vi "ws_configure restart dynamic.vi"() -> ()   [LabVIEW 2011]
panel:
  in  "rendezvous":T1
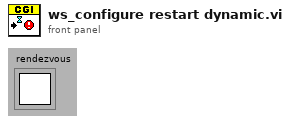
[diagram p1: front panel]
types:
  T1 = typedef "Rendezvous RefNum" = refnum<k1>
  T2 = typedef "Keyed Array.ctl" = cluster{"keys":string[], "values":string[]}
  T3 = enum32{"invalid app kind", "Development System", "Run Time System", "Student Edition", "Embedded LabVIEW", "Evaluation", "Custom"}
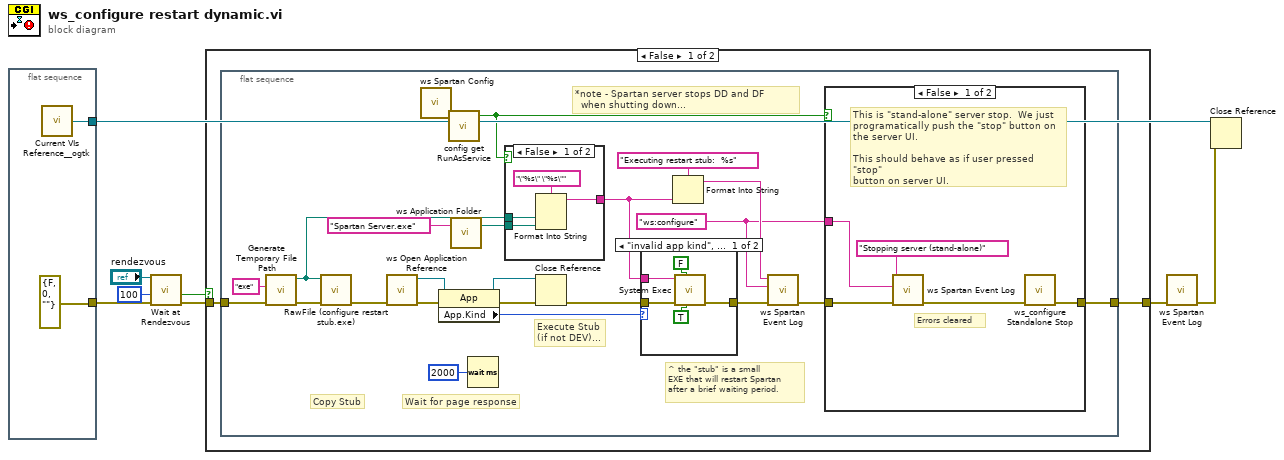
[diagram p0: block diagram]
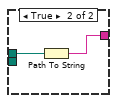
[diagram p2: hidden frame]
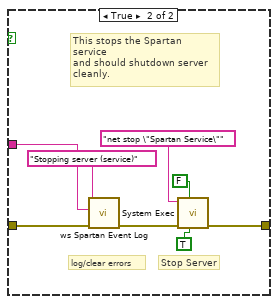
[diagram p4: hidden frame]
diagram:
  n1 = flat-sequence {
    tunnel: [w9] -> w3
    tunnel: [errorcluster {"status"=FALSE, "code"=0, "source"=""} ("error in (no error)")] -> w4
    frame #0 {
      n2 = call <userlib>:"Current VIs Reference__ogtk.vi"() -> ("Current VI's reference"=w9:refnum<vi>)  [unwired: 5 out]
    }
  }
  n3 = call <vilib>:"Wait at Rendezvous.vi"("error in (no error)"=w4, "ms timeout (-1)"=100, "rendezvous"="rendezvous") -> ("error out"=w6:errorcluster, "timed out"=w5:bool)  [unwired: 3 out]
  n4 = case shown="False" w5 {
    tunnel: [w12 w61] -> w2
    tunnel: w6 -> [w11 w61]
    frame False {
      n5 = flat-sequence {
        tunnel: [w35] -> w12
        tunnel: w11 -> [w19]
        frame #0 {
          w30 = "ws:configure" ("command line")
          # "Wait for page response"
          # "Copy Stub"
          # "*note - Spartan server stops DD and DF\n  when shutting down..."
          # "^ the \"stub\" is a small\nEXE that will restart Spartan\nafter a brief waiting period."
          # "Execute Stub\n(if not DEV)..."
          n6 = call <vilib>:"Generate Temporary File Path.vi"("error in (no error)"=w19, "Temporary File Extension (tmp)"="exe") -> ("error out"=w23:errorcluster, "Unique Temporary File Path"=w20:path)  [unwired: 8 out]
          n7 = call "RawFile (configure restart stub.exe).vi"("error in (no error)"=w23, "Path to File (empty)"=w20) -> ("error out"=w15:errorcluster)  [unwired: 9 out]
          n8 = call "ws Open Application Reference.vi"("error in (no error)"=w15) -> ("error out"=w14:errorcluster, "application reference"=w13:refnum<vi>)  [unwired: 9 in]
          n9 = call "ws Spartan Config.vi"() -> ("CONFIG"=w16:T2)  [unwired: 9 in, 2 out]
          n10 = property class="App"(reference=w13, error in=w14) -> (reference out=w25:refnum<vi>, error out=w26:errorcluster, "App.Kind"=w27:T3)
          n11 = call "config get RunAsService.vi"("Config Keys"=w16) -> ("RunAsService?"=w34:bool)  [unwired: 4 out]
          n12 = call "ws Application Folder.vi"("Relative Path (\"\" - Folder)"="Spartan Server.exe" ("command line")) -> ("Application Folder"=w17:path)  [unwired: 2 in]
          n13 = Wait (ms)(milliseconds to wait=u32 2000) -> ()  [unwired: 1 out]
          n14 = case shown="False" w34 {
            tunnel: [w38 w40] -> w31
            tunnel: w20 -> [w37 w41]
            tunnel: w17 -> [w36 _]
            frame False {
              n15 = Format Into String(format string="\"%s\" \"%s\"", w37, w36) -> (resulting string=w38:string)  [unwired: 2 in, 1 out]
            }
            frame True {
              n16 = Path To String(path=w41) -> (string=w40:string)
            }
          }
          n17 = Close Reference(reference=w25, error in (no error)=w26) -> (error out=w24:errorcluster)
          n18 = case shown="\"invalid app kind\", Default" w27 {
            tunnel: w24 -> [w44 w47]
            tunnel: [w43 w47] -> w29
            tunnel: w31 -> [w42 _]
            frame "invalid app kind", Default {
              n19 = call <vilib>:"System Exec.vi"("run minimized? (F)"=TRUE, "wait until completion? (T)"=FALSE, "error in (no error)"=w44, "command line"=w42) -> ("error out"=w43:errorcluster)  [unwired: 2 in, 5 out]
            }
            frame "Development System" {
            }
          }
          n20 = Format Into String(format string="Executing restart stub:  %s", w31) -> (resulting string=w32:string)  [unwired: 2 in, 1 out]
          n21 = call "ws Spartan Event Log.vi"("error in (no error)"=w29, "module (\"\")"=w30, "message (\"\")"=w32) -> ("error out"=w28:errorcluster)  [unwired: 5 in]
          n22 = case shown="False" w34 {
            tunnel: w28 -> [w52 w53]
            tunnel: [w48 w58] -> w35
            tunnel: w30 -> [w51 w54]
            frame False {
              # "Errors cleared"
              # "This is \"stand-alone\" server stop.  We just\nprogramatically push the \"stop\" button on\nthe server UI.\n\nThis should behave as if user pressed \"stop\"\nbutton on server UI."
              n23 = call "ws Spartan Event Log.vi"("error in (no error)"=w52, "module (\"\")"=w51, "message (\"\")"="Stopping server (stand-alone)") -> ("error out"=w49:errorcluster)  [unwired: 5 in]
              n24 = call "ws_configure Standalone Stop.vi"("error in (no error)"=w49) -> ("error out"=w48:errorcluster)  [unwired: 6 in]
            }
            frame True {
              # "This stops the Spartan service\nand should shutdown server\ncleanly."
              # "Stop Server"
              # "log/clear errors"
              n25 = call "ws Spartan Event Log.vi"("error in (no error)"=w53, "module (\"\")"=w54, "message (\"\")"="Stopping server (service)") -> ("error out"=w56:errorcluster)  [unwired: 5 in]
              n26 = call <vilib>:"System Exec.vi"("run minimized? (F)"=TRUE, "wait until completion? (T)"=FALSE, "error in (no error)"=w56, "command line"="net stop \"Spartan Service\"") -> ("error out"=w58:errorcluster)  [unwired: 2 in, 5 out]
            }
          }
        }
      }
    }
    frame True {
    }
  }
  n27 = call "ws Spartan Event Log.vi"("error in (no error)"=w2) -> ("error out"=w1:errorcluster)  [unwired: 7 in]
  n28 = Close Reference(reference=w3, error in (no error)=w1) -> ()  [unwired: 1 out]
